vi "AdditionSubtraction.vi"() -> ()   [LabVIEW 2019]
panel:
  in  "Traditional DAQ Channel":tag
  in  "Tab Control":enum32{"Page 1", "Page 2"}(tab)
  out "Addition":dbl
  out "Subtraction":dbl
  out "MultiPlication":dbl
  out "Division":dbl
  in  "Ring":u16(ring) items=["", "kaanpuriya", "joseph Lee ", "sir Name"]
  in  "Second Number":dbl
  in  "First Number":dbl
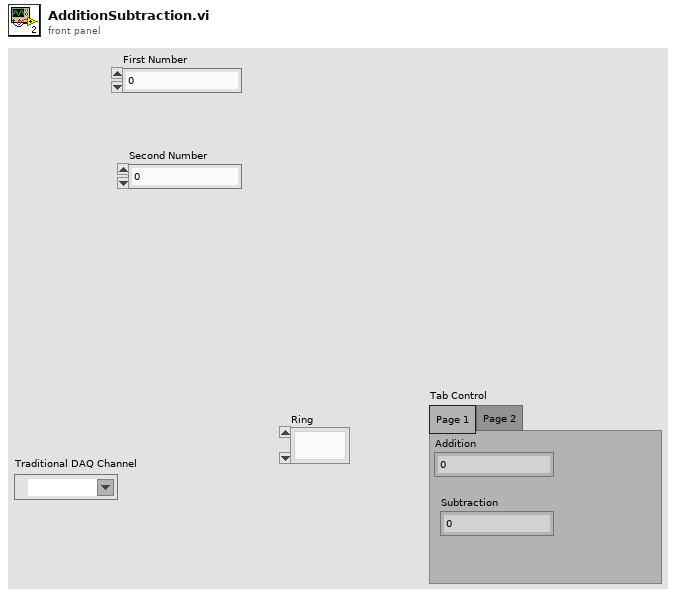
[diagram p1: front panel]
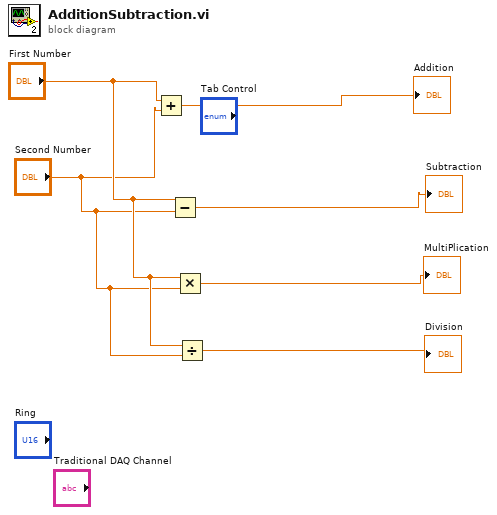
[diagram p0: block diagram]
diagram:
  n1 = Add(x="First Number", y="Second Number") -> (x+y=→"Addition":dbl)
  n2 = Subtract(x="First Number", y="Second Number") -> (x-y=→"Subtraction":dbl)
  n3 = Multiply(x="First Number", y="Second Number") -> (x*y=→"MultiPlication":dbl)
  n4 = Divide(x="First Number", y="Second Number") -> (x/y=→"Division":dbl)
